vi "Reset Device Core.vi"(8 "error in (no error)":errorcluster, 11 "IVI_Fgen in":refnum<class "IVI_Fgen.lvclass">) -> (0 "error out":errorcluster, 3 "IVI_Fgen out":refnum<class "IVI_Fgen.lvclass">)   [LabVIEW 2014, in "IVI_Fgen.lvlib" / "IVI_Fgen.lvclass"]
doc: "Perform reset of device."
uses:
  IVI_Fgen.lvclass
  CSPP_Core/Actors/CS++DeviceActor/CS++DeviceActor.lvclass/CS++DeviceActor.ctl
  IVI_Fgen.lvclass/IVI_Fgen.ctl
  CSPP_Core/Actors/CS++DeviceActor/CS++DeviceActor.lvclass
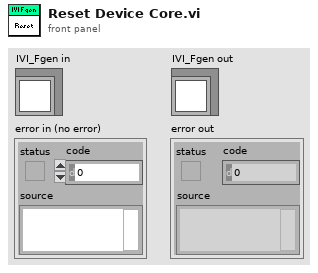
[diagram p1: front panel]
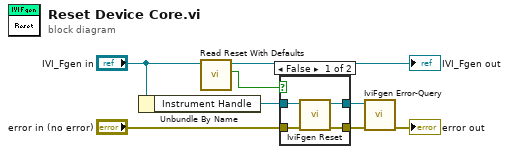
[diagram p0: block diagram]
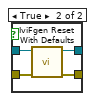
[diagram p2: hidden frame]
diagram:
  n1 = Unbundle By Name("IVI_Fgen in") -> ("Instrument Handle"=w8:refnum<k15>)
  n2 = call "Read Reset With Defaults.vi"("CS++DeviceActor in"="IVI_Fgen in") -> ("Reset With Defaults"=w1:bool, "CS++DeviceActor out"=→"IVI_Fgen out":refnum<class "IVI_Fgen.lvclass">)  [unwired: 8 in, 1 out]
  n3 = case shown="False" w1 {
    tunnel: w8 -> [w11 w16]
    tunnel: "error in (no error)" -> [w12 w15]
    tunnel: [w10 w14] -> w6
    tunnel: [w9 w13] -> w5
    frame False {
      n4 = call <vilib>:"IviFgen Reset.vi"("error in (no error)"=w12, "instrument handle"=w11) -> ("error out"=w10:errorcluster, "instrument handle out"=w9:refnum<k15>)  [unwired: 8 in]
    }
    frame True {
      n5 = call <vilib>:"IviFgen Reset With Defaults.vi"("error in (no error)"=w15, "instrument handle"=w16) -> ("error out"=w14:errorcluster, "instrument handle out"=w13:refnum<k15>)  [unwired: 8 in]
    }
  }
  n6 = call <vilib>:"IviFgen Error-Query.vi"("error in (no error)"=w6, "instrument handle"=w5) -> ("error out"=→"error out":errorcluster)  [unwired: 6 in, 3 out]
